vi "数据库查询.vi"() -> (2 "查询结果":string[][](table))   [LabVIEW 2010]
panel:
  in  "error in (no error) 2":errorcluster caption="错误输入（无错误）"
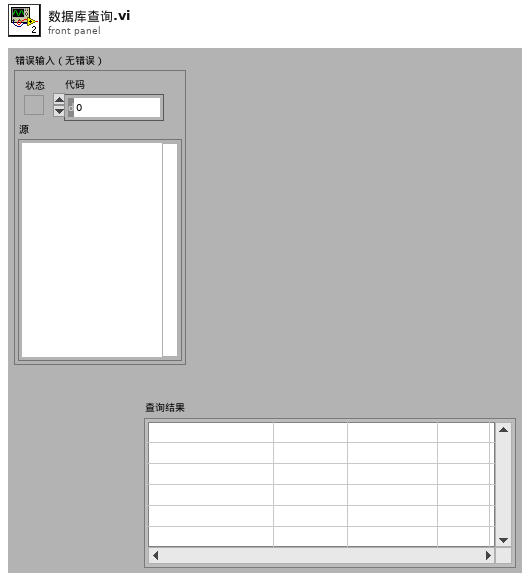
[diagram p1: front panel]
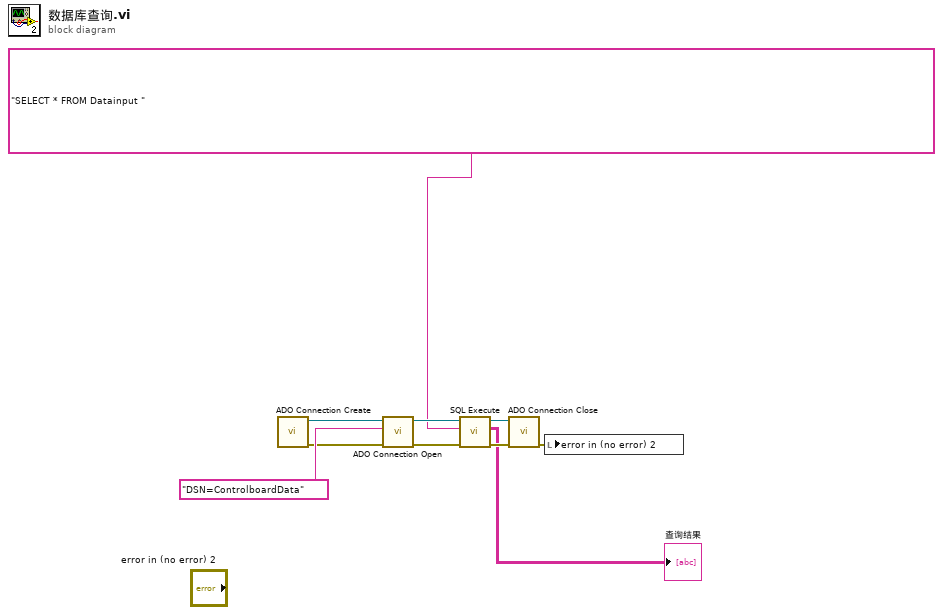
[diagram p0: block diagram]
diagram:
  n1 = call "ADO Connection Create.vi"() -> ("error out"=w4:errorcluster, "ADODB._Connection Out"=w3:refnum<k7>)  [unwired: 10 in]
  n2 = call "ADO Connection Open.vi"("error in (no error)"=w4, "ConnectionString"="DSN=ControlboardData", "ADODB._Connection In"=w3) -> ("error out"=w7:errorcluster, "ADODB._Connection Out"=w10:refnum<k7>)  [unwired: 7 in]
  n3 = call "SQL Execute.vi"("error in (no error)"=w7, "Command Text"="SELECT * FROM Datainput ", "ADODB._Connection In"=w10) -> ("error out"=w6:errorcluster, "Data"=→"查询结果":string[][], "ADODB._Connection Out"=w9:refnum<k7>)  [unwired: 5 in, 1 out]
  n4 = call "ADO Connection Close.vi"("error in (no error)"=w6, "ADODB._Connection In"=w9) -> ("error out"=w5:errorcluster)  [unwired: 8 in, 1 out]
  n5 = local write "error in (no error) 2"(w5) -> ()
